vi "set_shutter.vi"(8 "error in (no error)":errorcluster, 10 "shutter open?":bool=TRUE, 11 "LightSourceMH110124MaiTai in":refnum<class "LightSourceMH110124MaiTai.lvclass">) -> (0 "error out":errorcluster, 2 "shutter open out?":bool, 3 "LightSourceMH110124MaiTai out":refnum<class "LightSourceMH110124MaiTai.lvclass">)   [LabVIEW 2010, in "LightSourceMH110124MaiTai.lvclass"]
uses:
  LightSourceMH110124MaiTai.lvclass
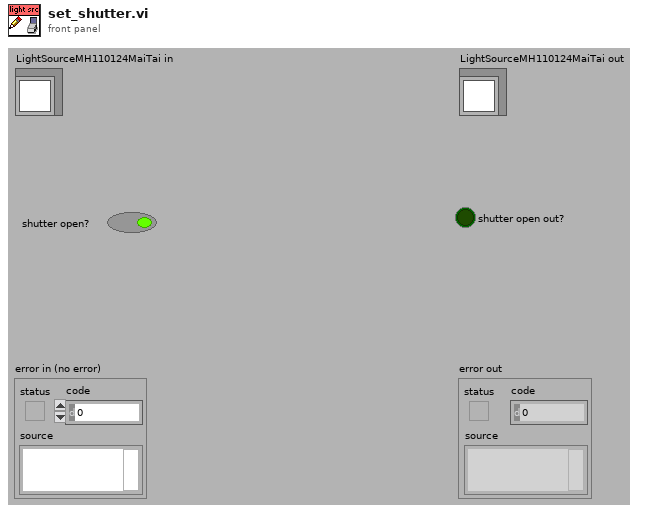
[diagram p1: front panel]
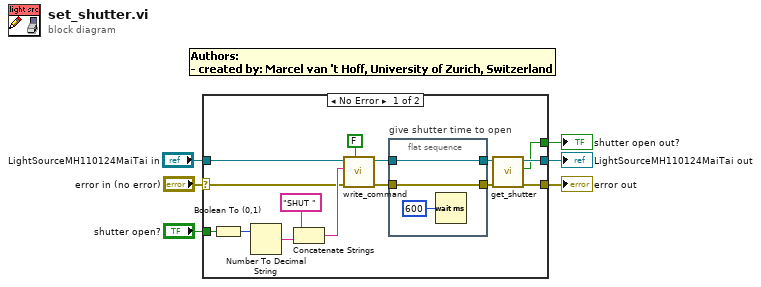
[diagram p0: block diagram]
diagram:
  n1 = case shown="No Error" "error in (no error)" {
    selector: "error in (no error)" -> [w7 w26]
    tunnel: [w16 w26] -> w4
    tunnel: [w15 w25] -> w5
    tunnel: "LightSourceMH110124MaiTai in" -> [w8 w25]
    tunnel: "shutter open?" -> [w21 _]
    tunnel: [w13 _] -> w1
    frame No Error {
      n2 = Boolean To (0,1)(Boolean=w21) -> (0, 1=w20:i16)
      n3 = Number To Decimal String(number=w20) -> (decimal integer string=w19:string)  [unwired: 1 in]
      n4 = Concatenate Strings("SHUT ", w19) -> (w17:string)
      n5 = call-dynamic "write_command.vi"("read (T)"=FALSE, "error in (no error)"=w7, "string to write"=w17, "LightSourceMH110124MaiTai in"=w8) -> ("error out"=w11:errorcluster, "LightSourceMH110124MaiTai out"=w12:refnum<class "LightSourceMH110124MaiTai.lvclass">)  [unwired: 5 in, 1 out]
      n6 = flat-sequence "give shutter time to open" {
        tunnel: w12 -> [w23]
        tunnel: w11 -> [w24]
        tunnel: [w24] -> w10
        tunnel: [w23] -> w9
        frame #0 {
          n7 = Wait (ms)(milliseconds to wait=u32 600) -> ()  [unwired: 1 out]
        }
      }
      n8 = call-dynamic "get_shutter.vi"("error in (no error)"=w10, "LightSourceMH110124MaiTai in"=w9) -> ("error out"=w16:errorcluster, "shutter open out?"=w13:bool, "LightSourceMH110124MaiTai out"=w15:refnum<class "LightSourceMH110124MaiTai.lvclass">)  [unwired: 7 in]
    }
    frame Error {
    }
  }
  "error out" <- w4
  "LightSourceMH110124MaiTai out" <- w5
  "shutter open out?" <- w1
